vi "GetObjectStatus.vi"(0 "reference in":refnum<class "IG#.lvclass">, 2 "simple info (F)":bool, 5 "error in (no error)":errorcluster) -> (8 "full class name":string, 9 "# of users?":i32, 10 "all object names":string[](array[string]), 11 "last user":bool, 12 "# of objects":i32, 13 "class name":string, 14 "reference out":refnum<class "IG#.lvclass">, 15 "not a refnum?":bool, 16 "object name":string, 17 "all refs out":refnum<class "G#Object.lvclass">[](array[class]), 18 "counter?":bool, 19 "error out":errorcluster)   [LabVIEW 2020, in "IG#.lvclass"]
doc: "Returns information about the specified object. If simple info = true, only object info is return and not the arrays of objects.\n\nIf input reference is invalid, only information about the class is returned."
uses:
  IG#.lvclass
  G#Object/G#Object.lvclass
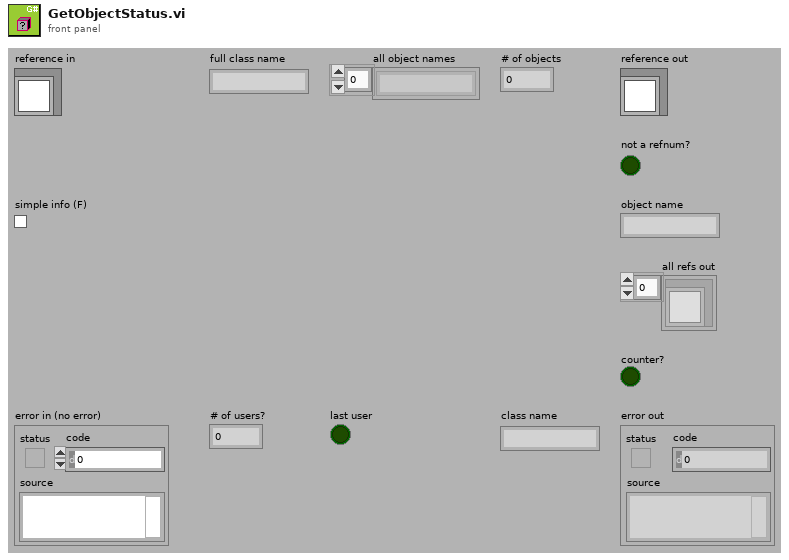
[diagram p1: front panel]
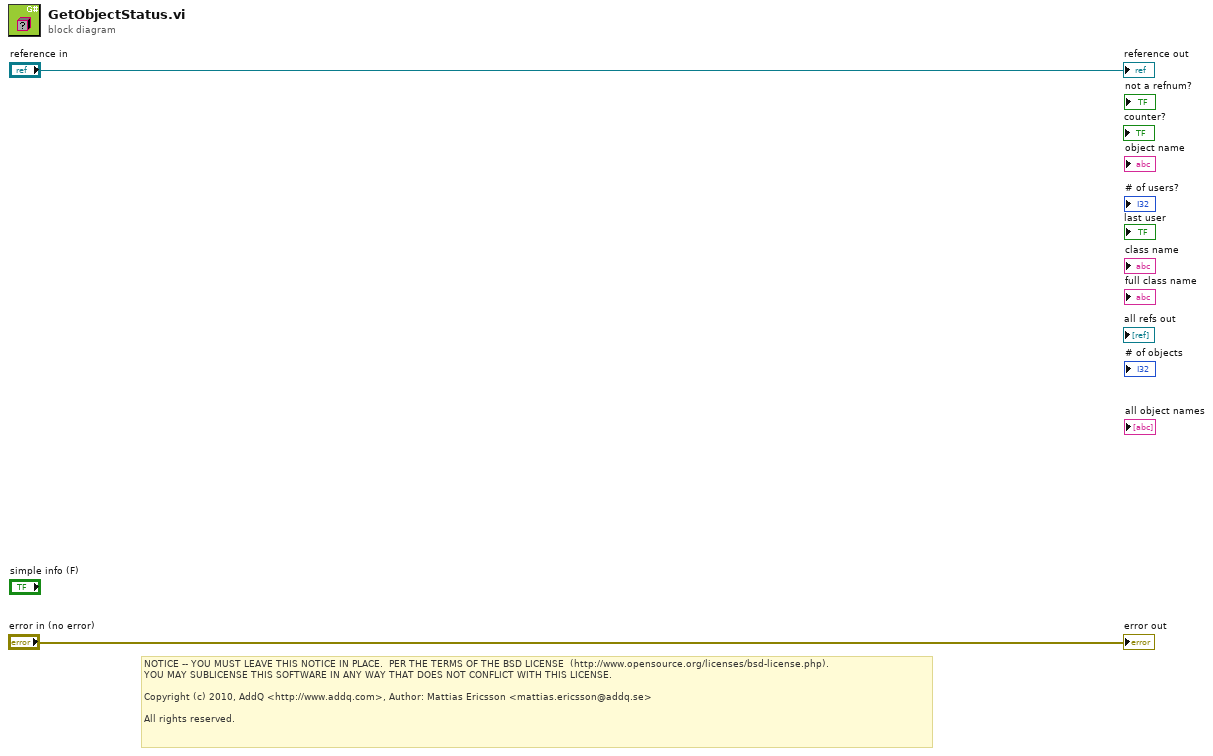
[diagram p0: block diagram]
diagram:
  # "NOTICE -- YOU MUST LEAVE THIS NOTICE IN PLACE.  PER THE TERMS OF THE BSD LICENSE  (http://www.opensource.org/licenses/bsd-license.php).\nYOU MAY SUBLICENSE THIS SOFTWARE IN ANY WAY THAT DOES NOT CONFLICT WITH THIS LICENSE.\n\nCopyright (c) 2010, AddQ <http://www.addq.com>, Author: Mattias Ericsson <mattias.ericsson@addq.se>\n\nAll rights reserved."
  "reference out" <- "reference in"
  "error out" <- "error in (no error)"
